vi "Write Context.vi"(8 "error in (no error)":errorcluster, 10 "Context":T1={"Continue Test"=FALSE, "DUT Info"={"SN"="", "Model"="", "PartNumber"="", "Revision"="", "Software"="", "Hardware"=""}, "StartTime"=timestamp(0 s since 1904-01-01), "EndTime"=timestamp(0 s since 1904-01-01), "Result"=enum."Terminated", "Info Text"="", "ResultList"=[]}, 11 "Execution in":refnum<class "Execution.lvclass">) -> (0 "error out":errorcluster, 3 "Execution out":refnum<class "Execution.lvclass">)   [LabVIEW 2015, in "Execution.lvclass"]
uses:
  Execution.lvclass
  EXECUTION_CONTEXT.ctl
  DUT_INFO_TYPEDEF.ctl
  EXECUTION_RESULT_TYPEDEF.ctl
  STEP_RESULT.ctl
  Step.lvclass
  Step/STEP_STATUS.ctl
  STEP_MEASURE_RESULT.ctl
  Step/OUTPUT_DATA_TYPE.ctl
  OutputUI/OUTPUT_CHECK_TYPE.ctl
  Execution.lvclass/Execution.ctl
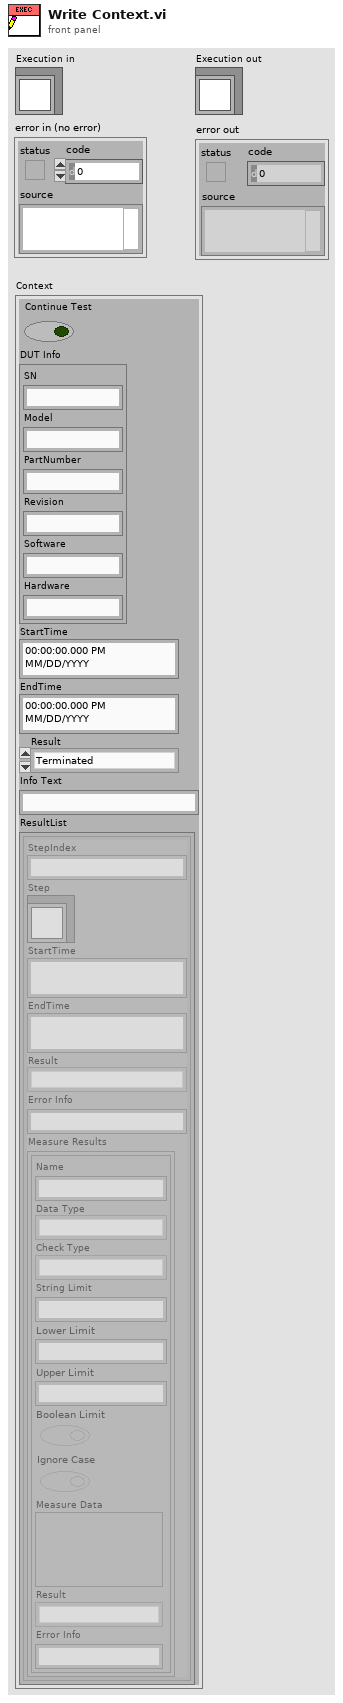
[diagram p1: front panel]
types:
  T1 = typedef "Execution.lvclass/EXECUTION_CONTEXT.ctl" = cluster{"Continue Test":bool, "DUT Info":T2, "StartTime":timestamp, "EndTime":timestamp, "Result":T3, "Info Text":string, "ResultList":T4[]}
  T2 = typedef "Execution.lvclass/DUT_INFO_TYPEDEF.ctl" = cluster{"SN":string, "Model":string, "PartNumber":string, "Revision":string, "Software":string, "Hardware":string}
  T3 = typedef "Execution.lvclass/EXECUTION_RESULT_TYPEDEF.ctl" = enum16{"Unknow", "Terminated", "Passed", "Failed", "Error"}
  T4 = typedef "Execution.lvclass/STEP_RESULT.ctl" = cluster{"StepIndex":u32, "Step":refnum<class "Step.lvclass">, "StartTime":timestamp, "EndTime":timestamp, "Result":T5, "Error Info":string, "Measure Results":T6[]}
  T5 = typedef "Step.lvclass/STEP_STATUS.ctl" = enum16{"Skipped", "Done", "Passed", "Failed", "Error"}
  T6 = typedef "Execution.lvclass/STEP_MEASURE_RESULT.ctl" = cluster{"Name":string, "Data Type":T7, "Check Type":T8, "String Limit":string, "Lower Limit":dbl, "Upper Limit":dbl, "Boolean Limit":bool, "Ignore Case":bool, "Measure Data":variant, "Result":T5, "Error Info":string}
  T7 = typedef "Step.lvclass/OUTPUT_DATA_TYPE.ctl" = enum16{"Boolean", "String", "Numeric", "Other"}
  T8 = typedef "Step.lvclass/OUTPUT_CHECK_TYPE.ctl" = enum16{"INVALID", "DO_NOT_CHECK", "RECORD", "VARIABLE", "EQUAL", "NOT_EQUAL", "STR_CONTAINS", "STR_START_WITH", "STR_END_WITH", "STR_REGEX_MATCH", "NUM_GT", "NUM_LT", "NUM_GE", "NUM_LE", "NUM_RANGE", "NUM_RANGE_BDY"}
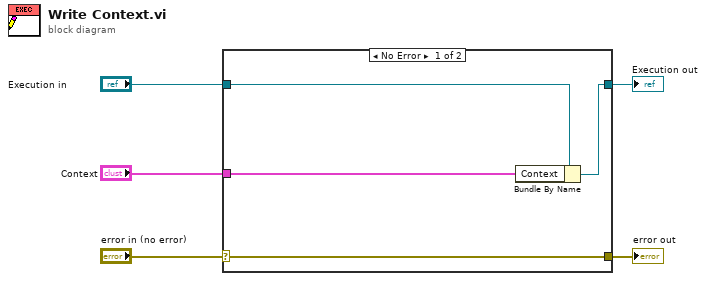
[diagram p0: block diagram]
diagram:
  n1 = case shown="No Error" "error in (no error)" {
    selector: "error in (no error)" -> [w9 w10]
    tunnel: [w9 w10] -> w4
    tunnel: [w7 w11] -> w2
    tunnel: "Execution in" -> [w8 w11]
    tunnel: "Context" -> [w6 _]
    frame No Error {
      n2 = Bundle By Name(cluster=w8, "Context"=w6) -> (w7:refnum<class "Execution.lvclass">)
    }
    frame Error {
    }
  }
  "error out" <- w4
  "Execution out" <- w2
